vi "CoordinateConvert_ShoulderOriginCartesianToWorldCartesian_Array.vi"(1 "ArmPositionRelativeToShoulderIn":T1[](array[typedef]), 2 "RobotDimensions":T2) -> (0 "ArmAbsolutePosition":T1[](array[typedef]))   [LabVIEW 2018]
uses:
  TypeDefs/ConfigComponents/Config_Dimensions.ctl
  TypeDefs/ArmAbsolutePosition.ctl
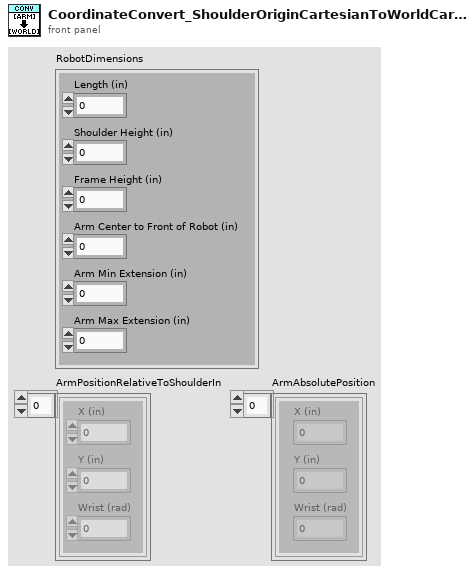
[diagram p1: front panel]
types:
  T1 = typedef "ArmAbsolutePosition.ctl" = cluster{"X (in)":dbl, "Y (in)":dbl, "Wrist (rad)":dbl}
  T2 = typedef "Config_Dimensions.ctl" = cluster{"Length (in)":dbl, "Shoulder Height (in)":dbl, "Frame Height (in)":dbl, "Arm Center to Front of Robot (in)":dbl, "Arm Min Extension (in)":dbl, "Arm Max Extension (in)":dbl}
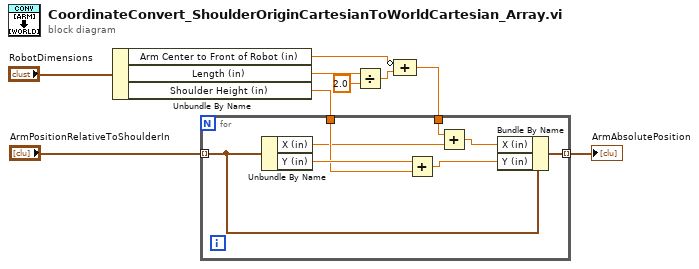
[diagram p0: block diagram]
diagram:
  n1 = Unbundle By Name("RobotDimensions") -> ("Arm Center to Front of Robot (in)"=w6:dbl, "Length (in)"=w8:dbl, "Shoulder Height (in)"=w4:dbl)
  n2 = Divide(x=w8, y=2.0) -> (x/y=w5:dbl)
  n3 = Compound Arithmetic op=ADD(invert w6, w5) -> (w3:dbl)
  n4 = for {
    tunnel: w4 -> [w16]
    tunnel: w3 -> [w14]
    tunnel: "ArmPositionRelativeToShoulderIn" -> [w11] mode=indexing
    tunnel: [w10] -> w1 mode=indexing
    n5 = Unbundle By Name(w11) -> ("X (in)"=w13:dbl, "Y (in)"=w17:dbl)
    n6 = Add(x=w17, y=w16) -> (x+y=w15:dbl)
    n7 = Add(x=w14, y=w13) -> (x+y=w12:dbl)
    n8 = Bundle By Name(cluster=w11, "X (in)"=w12, "Y (in)"=w15) -> (w10:T1)
  }
  "ArmAbsolutePosition" <- w1
